vi "to string.vi"(8 "error in":errorcluster, 11 "engine configuration in":refnum<class "base TBM sequencer configuration.lvclass">) -> (0 "error out":errorcluster, 1 "data":string, 2 "version":string, 3 "engine configuration out":refnum<class "base TBM sequencer configuration.lvclass">)   [LabVIEW 2014, in "base TBM sequencer configuration.lvclass"]
doc: "This VI takes an Engine Configuration object and flattens it into a string with corresponding version. The version is used that the data string can be unflattenend successfully as the configuration object evolves over time."
uses:
  base TBM sequencer configuration.lvclass
  Version Constant.vi
  <vilib>/NI/Tag Bus Module Framework/module configuration/TBM module configuration.lvclass
  <vilib>/NI/Configuration Framework/serializable configuration/NISE_CEF_serializable configuration.lvclass
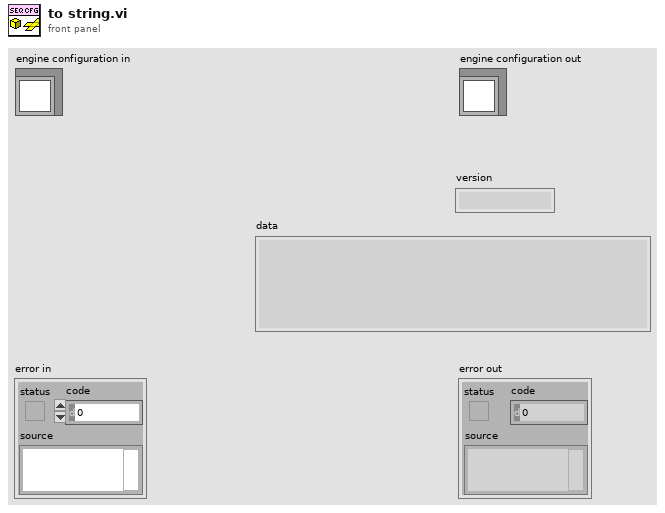
[diagram p1: front panel]
types:
  T1 = typedef "base TBM sequencer configuration.lvclass/Module Mappings.ctl" = cluster{"Owning ID":string, "Input Mappings":T2[], "Process Parameter Mappings":T2[], "Process Results Mappings":T2[], "Output Mappings":T2[]}
  T2 = typedef "tag bus.lvlib/data table.lvlib/mapping specification.ctl" = cluster{"data type":T3, "mappings":T4[]}
  T3 = typedef "tag bus.lvlib/tag descriptor.lvclass/Data Type.ctl" = enum16{"Double", "Single", "I64", "I32", "I16", "I8", "U64", "U32", "U16", "U8", "Boolean", "String", "Array of Double", "Array of Single", "Array of I64", "Array of I32", "Array of I16", "Array of I8", "Array of U64", "Array of U32", "Array of U16", "Array of U8", "Array of Boolean", "Array of String"}
  T4 = typedef "tag bus.lvlib/data table.lvlib/mapping.ctl" = cluster{"sink name":string, "source name":string}
  T5 = typedef "base TBM sequencer configuration.lvclass/Tag Info.ctl" = cluster{"Channel":refnum<class "TBM channel.lvclass">, "Writers":string[], "Readers":string[], "Owning ID":string}
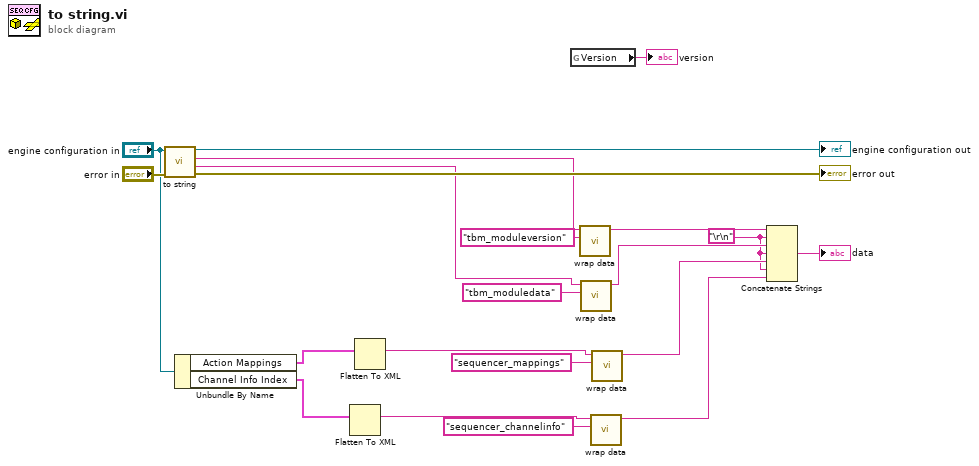
[diagram p0: block diagram]
diagram:
  w2 = "\r\n"
  n1 = call-parent "to string.vi"("error in"="error in", "module configuration in"="engine configuration in") -> ("error out"=→"error out":errorcluster, "data"=w13:string, "version"=w14:string, "module configuration out"=→"engine configuration out":refnum<class "base TBM sequencer configuration.lvclass">)  [unwired: 6 in]
  n2 = Unbundle By Name("engine configuration in") -> ("Action Mappings"=w6:T1[], "Channel Info Index"=w5:T5[])
  n3 = Flatten To XML(anything=w5) -> (xml string=w3:string)
  n4 = Flatten To XML(anything=w6) -> (xml string=w4:string)
  n5 = global read "Version Constant.vi" "Version"() -> (→"version":string)
  n6 = call <vilib>:"wrap data.vi"("identifier"="tbm_moduleversion" ("additional identifier"), "data to wrap"=w14) -> ("wrapped data"=w15:string)  [unwired: 9 in]
  n7 = call <vilib>:"wrap data.vi"("identifier"="tbm_moduledata" ("additional identifier"), "data to wrap"=w13) -> ("wrapped data"=w16:string)  [unwired: 9 in]
  n8 = call <vilib>:"wrap data.vi"("identifier"="sequencer_channelinfo" ("additional identifier"), "data to wrap"=w3) -> ("wrapped data"=w7:string)  [unwired: 9 in]
  n9 = call <vilib>:"wrap data.vi"("identifier"="sequencer_mappings" ("additional identifier"), "data to wrap"=w4) -> ("wrapped data"=w8:string)  [unwired: 9 in]
  n10 = Concatenate Strings(w15, w2, w16, w2, w8, w2, w7) -> (→"data":string)
